vi "Search Bookmarks with event names Requests.vi"(8 "error in":errorcluster, 9 "Request":string, 10 "VIs to Search for Bookmarks Paths":path[](array[path]), 11 "Application in":refnum<vi>) -> (0 "error out":errorcluster)   [LabVIEW 2016, in "PantherLAB_Scripting.lvlib"]
uses:
  PantherLAB_Scripting.lvlib
  <vilib>/Utility/traverseref.llb/TRef TravTarget.ctl
  <vilib>/Utility/traverseref.llb/VI Scripting - Traverse.lvlib
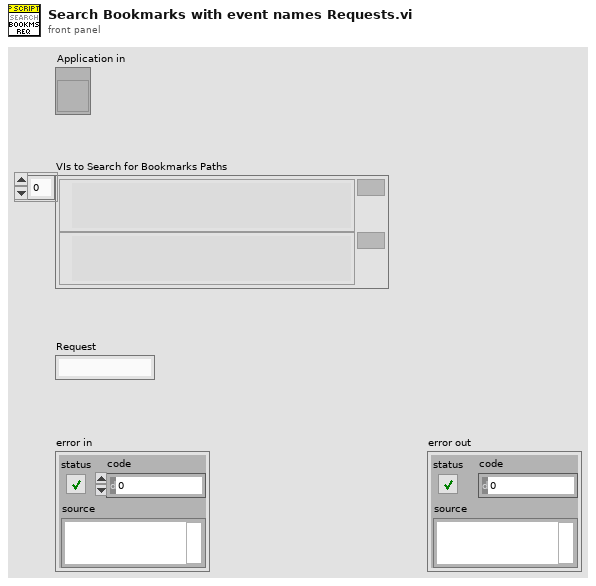
[diagram p1: front panel]
types:
  T1 = typedef "TRef TravTarget.ctl" = enum16{"FP", "BD", "Other"}
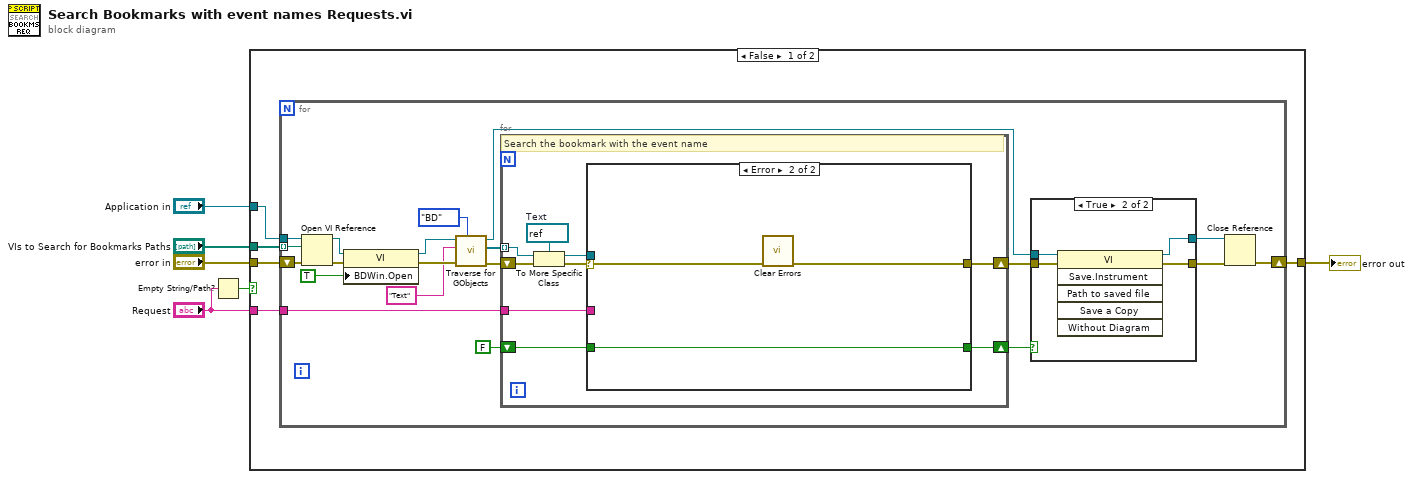
[diagram p0: block diagram]
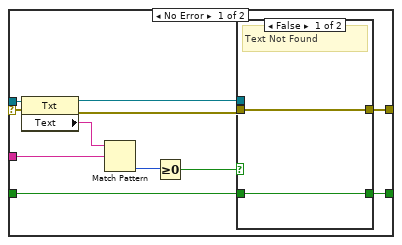
[diagram p2: hidden frame]
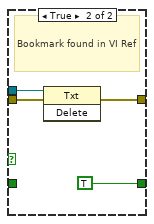
[diagram p3: hidden frame]
diagram:
  n1 = Empty String/Path?(string/path="Request") -> (empty?=w1:bool)
  n2 = case shown="False" w1 {
    tunnel: [w11 w67] -> w6
    tunnel: "error in" -> [w10 w67]
    tunnel: "Request" -> [w9 _]
    tunnel: "Application in" -> [w8 _]
    tunnel: "VIs to Search for Bookmarks Paths" -> [w7 _]
    frame False {
      n3 = for {
        tunnel: w8 -> [w19]
        tunnel: w7 -> [w17] mode=indexing
        shift-right: [w26] -> w11
        shift-left: w10 -> [w27]
        tunnel: w9 -> [w12]
        n4 = Open VI Reference(application reference (local)=w19, vi path=w17, error in (no error)=w27) -> (vi reference=w21:refnum<vi>, error out=w29:errorcluster)  [unwired: 3 in]
        n5 = property class="VI"(reference=w21, error in=w29, "BDWin.Open"=TRUE ("Block Diagram Window:Open")) -> (reference out=w20:refnum<vi>, error out=w28:errorcluster)
        n6 = call <vilib>:"Traverse for GObjects.vi"("Traverse Target"=TRef_TravTarget."BD", "error in (no error)"=w28, "Class Name"="Text", "VI Refnum"=w20) -> ("error out"=w31:errorcluster, "References"=w18:refnum<vi>[], "dup VI Refnum"=w15:refnum<vi>)  [unwired: 4 in, 1 out]
        n7 = for {
          shift-right: [w39] -> w30
          shift-left: w31 -> [w40]
          tunnel: w18 -> [w36] mode=indexing
          shift-right: [w33] -> w13
          shift-left: FALSE -> [w34]
          tunnel: w12 -> [w32]
          w37 = refnum<vi> refnum  # Text
          # "Search the bookmark with the event name"
          n8 = To More Specific Class(target class=w37, reference=w36, error in=w40) -> (specific class reference=w35:refnum<vi>, error out=w38:errorcluster)
          n9 = case shown="Error" w38 {
            selector: w38 -> [w50 w60]
            tunnel: [w51 w58] -> w39
            tunnel: w35 -> [w48 _]
            tunnel: w34 -> [w45 w59]
            tunnel: [w44 w59] -> w33
            tunnel: w32 -> [w42 _]
            frame No Error {
              n10 = property class="Txt"(reference=w48, error in=w50) -> (reference out=w46:refnum<vi>, error out=w49:errorcluster, "Text"=w47:string)
              n11 = Match Pattern(string=w47, regular expression=w42) -> (offset past match=w43:i32)  [unwired: 1 in, 3 out]
              n12 = Greater Or Equal To 0?(x=w43) -> (x >= 0?=w41:bool)
              n13 = case shown="False" w41 {
                tunnel: w49 -> [w53 w57]
                tunnel: w46 -> [_ w55]
                tunnel: [w53 w56] -> w51
                tunnel: w45 -> [w52 _]
                tunnel: [w52 TRUE] -> w44
                frame False {
                  # "Text Not Found"
                }
                frame True {
                  # "Bookmark found in VI Ref"
                  n14 = invoke class="Txt" method="Delete"(reference=w55, error in=w57) -> (error out=w56:errorcluster)  [unwired: 1 in, 2 out]
                }
              }
            }
            frame Error {
              n15 = call <vilib>:"Clear Errors.vi"("error in (no error)"=w60) -> ("error out"=w58:errorcluster)  [unwired: 5 in, 1 out]
            }
          }
        }
        n16 = case shown="True" w13 {
          tunnel: w30 -> [w62 w66]
          tunnel: [w62 w65] -> w25
          tunnel: w15 -> [w61 w64]
          tunnel: [w61 w63] -> w14
          frame False {
          }
          frame True {
            n17 = invoke class="VI" method="Save.Instrument"(reference=w64, error in=w66) -> (reference out=w63:refnum<vi>, error out=w65:errorcluster)  [unwired: 4 in, 4 out]
          }
        }
        n18 = Close Reference(reference=w14, error in (no error)=w25) -> (error out=w26:errorcluster)
      }
    }
    frame True {
    }
  }
  "error out" <- w6
